vi "7-1 generatore di funzioni e multimetro.vi"(0 "n° byte rd":i32=30, 1 "rd delay":u32, 2 "cmd fun vet":string[](array[string])=["*cls", "", "", "appl:sin 100 HZ, 1 VPP"], 3 "cmd mult vet":string[](array[string])=["*cls", "conf:volt:ac 10, 0.001"], 4 "mode":i16) -> (5 "Tensione":dbl format="%.8f", 6 "Vout string":string)   [LabVIEW 2012]
doc: "© Copyright M. Ferrari 2000\nMisura singola Vac con HP34401A"
panel:
  out "status 4":bool
  out "after reading":i32
  out "status 3":bool
  out "read":i32
  out "status 2":bool
  out "iniz. gen.":i32
  out "status":bool
  out "code":i32
  in  "GPIB address Multimeter":string="4"
  in  "GPIB address Generator":string="10"
  # "PROPOSTA di SVILUPPO:\n\n1-  inviare le stringhe di configurazione al multimetro\n     inviare le stringhe per la selezione e la generazione della\n     forma d'onda voluta al generatore di funzioni\n\n2 -  inserire il ritardo programmabile\n\n3 -  effettuare la misura (multimetro) e riportare il valore\n      sul pannello  frontale del VI"
  # "Generator"
  # "Multimeter"
  # "sour:func:shap sin\n:freq 100 hz\n:volt 5 vpp\n\nappl:sin 100 HZ, 1 VPP"
  # "[sec]"
  # "MISURA SINGOLA CON GENERATORE di FUNZIONI HP33120A e MULTIMETRO HP34401A \n    Realizzare un VI che svolga le seguenti funzioni: \n   - configura il multimetro per una misura di tensione su un segnale, prodotto dal generatore \n     di funzioni, con le caratteristiche sotto riportate \n   - configura il generatore di funzioni in modo che generi una sinusoide con ampiezza di \n     1 volt (Vpp) alla frequenza di 100 Hz\n   - dopo un ritardo variabile (controllabile da pannello), effettua una misura, riportando il valore \n     letto dal multimetro su un indicatore apposito"
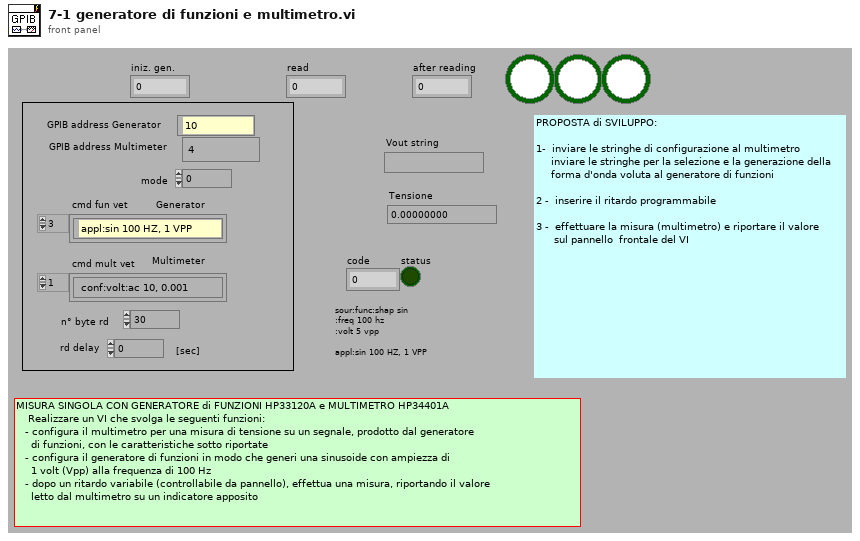
[diagram p1: front panel]
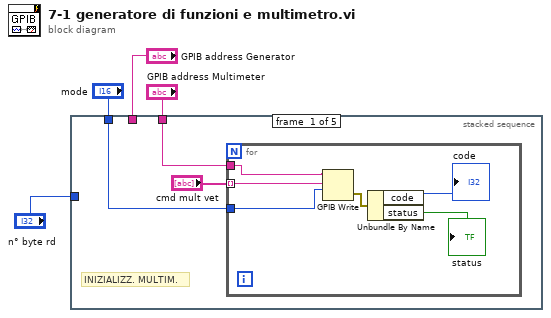
[diagram p0: block diagram]
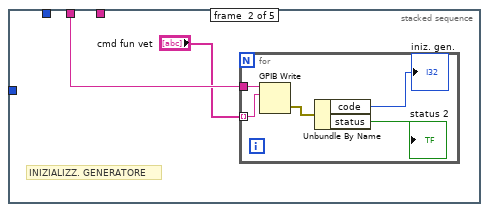
[diagram p2: hidden frame]
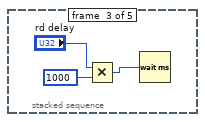
[diagram p3: hidden frame]
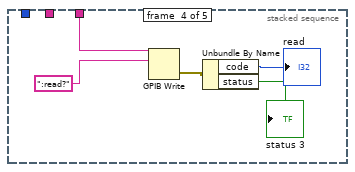
[diagram p4: hidden frame]
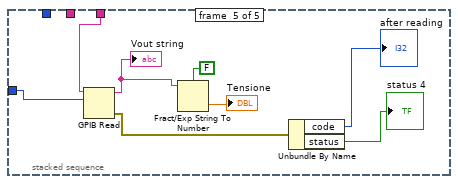
[diagram p5: hidden frame]
diagram:
  n1 = stacked-sequence {
    tunnel: "GPIB address Multimeter" -> [w7 _ _ w25 w33]
    tunnel: "mode" -> [w6 _ _ _ _]
    tunnel: "n° byte rd" -> [_ _ _ _ w34]
    tunnel: "GPIB address Generator" -> [_ w15 _ _ _]
    frame #0 {
      # "INIZIALIZZ. MULTIM."
      n2 = for {
        tunnel: w7 -> [w10]
        tunnel: "cmd mult vet" -> [w8] mode=indexing
        tunnel: w6 -> [w9]
        n3 = GPIB Write(0:w10, 1:w8, 2:w9) -> (6:w11:errorcluster)  [unwired: 2 in, 1 out]
        n4 = Unbundle By Name(w11) -> ("code"=→"code":i32, "status"=→"status":bool)
      }
    }
    frame #1 {
      # "INIZIALIZZ. GENERATORE"
      n5 = for {
        tunnel: w15 -> [w17]
        tunnel: "cmd fun vet" -> [w16] mode=indexing
        n6 = GPIB Write(0:w17, 1:w16) -> (6:w18:errorcluster)  [unwired: 3 in, 1 out]
        n7 = Unbundle By Name(w18) -> ("code"=→"iniz. gen.":i32, "status"=→"status 2":bool)
      }
    }
    frame #2 {
      n8 = Multiply(x="rd delay", y=u32 1000) -> (x*y=w21:u32)
      n9 = Wait (ms)(milliseconds to wait=w21) -> ()  [unwired: 1 out]
    }
    frame #3 {
      n10 = GPIB Write(0:w25, 1:":read?") -> (6:w27:errorcluster)  [unwired: 3 in, 1 out]
      n11 = Unbundle By Name(w27) -> ("code"=→"read":i32, "status"=→"status 3":bool)
    }
    frame #4 {
      n12 = GPIB Read(0:w33, 1:w34) -> (5:w32:string, 7:w29:errorcluster)  [unwired: 3 in, 1 out]
      "Vout string" <- w32
      n13 = Fract/Exp String To Number(use system decimal point (T)=FALSE, string=w32) -> (number=→"Tensione":dbl)  [unwired: 2 in, 1 out]
      n14 = Unbundle By Name(w29) -> ("code"=→"after reading":i32, "status"=→"status 4":bool)
    }
  }
